vi "SampleMethod.vi"(8 "error in (no error)":errorcluster, 11 "SampleLib in":refnum<class "SampleLib.lvclass">) -> (0 "error out":errorcluster, 3 "SampleLib out":refnum<class "SampleLib.lvclass">)   [LabVIEW 2019, in "SampleLibPPL.lvlib" / "SampleLib.lvclass"]
uses:
  SampleLib.lvclass
  SampleDependentLib.lvclass
  obj/SampleProjectTargets/My Computer/ExtDependency.lvlibp/ExternalDepClass/ExternalDepClass.lvclass
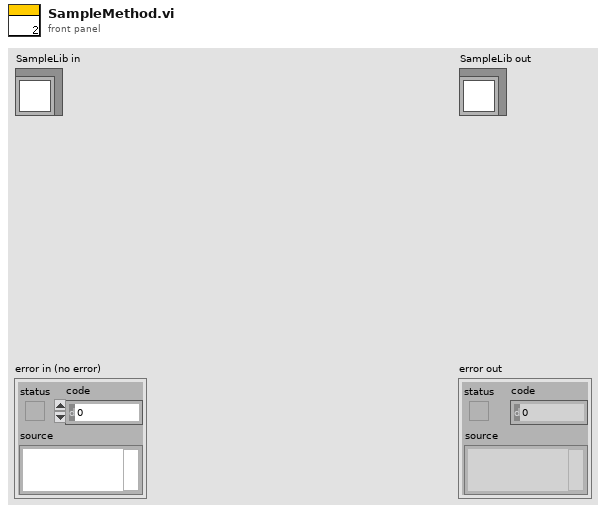
[diagram p1: front panel]
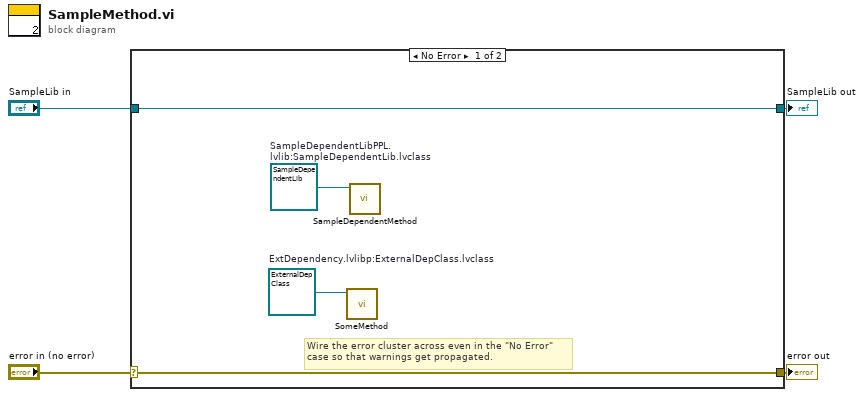
[diagram p0: block diagram]
diagram:
  n1 = case shown="No Error" "error in (no error)" {
    selector: "error in (no error)" -> [w7 w10]
    tunnel: [w7 w10] -> w3
    tunnel: [w8 w9] -> w1
    tunnel: "SampleLib in" -> [w8 w9]
    frame No Error {
      w5 = refnum<class "ExternalDepClass.lvclass"> refnum  # ExtDependency.lvlibp:ExternalDepClass.lvclass
      w6 = refnum<class "SampleDependentLib.lvclass"> refnum  # SampleDependentLibPPL.lvlib:SampleDependentLib.lvclass
      # "Wire the error cluster across even in the \"No Error\"\ncase so that warnings get propagated."
      n2 = call-dynamic "SomeMethod.vi"("ExternalDepClass in"=w5) -> ()  [unwired: 9 in, 2 out]
      n3 = call-dynamic "SampleDependentMethod.vi"("SampleDependentLib in"=w6) -> ()  [unwired: 9 in, 2 out]
    }
    frame Error {
    }
  }
  "error out" <- w3
  "SampleLib out" <- w1
